vi "(nist) Arm Globals.vi"() -> ()   [LabVIEW 2013]
panel:
  in  "L:Joints":dbl[](array[numeric])=[-0.416, -0.52, 1.12, -3.856, -0.084, -0.176, 0.14]
  in  "R:Joints":dbl[](array[numeric])=[-0.416, -0.52, 1.12, -3.856, -0.084, -0.176, 0.14]
  in  "R:Effort":dbl[](array[numeric])=[-0.416, -0.52, 1.12, -3.856, -0.084, -0.176, 0.14]
  # "Loaded from \nlabview_robotjoint_states_Server.vi\n(need to add \"(nist) Post Joint Values.vi\" to server)"
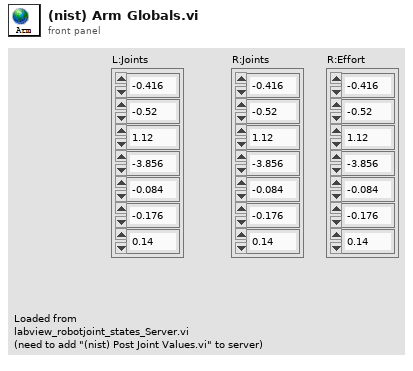
[diagram p1: front panel]
diagram:
